vi "CS SQL Server.queryOneStr.vi"(8 "error in (no error)":errorcluster, 10 "SQL query":string, 11 "connection reference":T1) -> (0 "error out":errorcluster, 1 "Query result":string, 3 "connection reference out":T1)   [LabVIEW 2014, in "CS SQL Server.lvlib"]
doc: "Thisa VI executes a SQL statement.\n\nIt is assumed that this quey expectes one element as result only!"
uses:
  CS SQL Server.lvlib
  <vilib>/addons/database/Connection.llb/Conn ObjectReference.ctl
  <vilib>/addons/database/Recordset.llb/Rec Destroy - Connection.vi
  <vilib>/addons/database/Recordset.llb/Rec Fetch Recordset Data (R).vi
  <vilib>/addons/database/Connection.llb/Conn Execute.vi
  <vilib>/addons/database/_DB Variant To Data/Database Variant To Data.xnode
  <vilib>/addons/database/NI_Database_API.lvlib
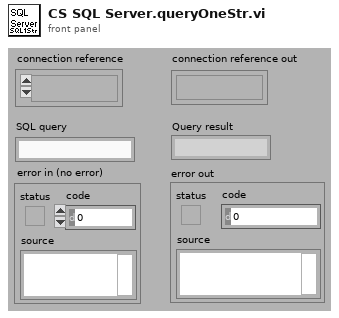
[diagram p1: front panel]
types:
  T1 = typedef "NI_Database_API.lvlib/Conn ObjectReference.ctl" = refnum<k1>
  T2 = typedef "NI_Database_API.lvlib/Rec ObjectReference.ctl" = refnum<k1>
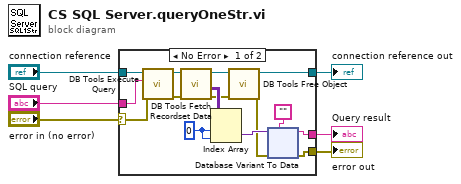
[diagram p0: block diagram]
diagram:
  n1 = case shown="No Error" "error in (no error)" {
    selector: "error in (no error)" -> [w7 w54]
    tunnel: "connection reference" -> [w12 w55]
    tunnel: "SQL query" -> [w11 _]
    tunnel: [w10 w55] -> w4
    tunnel: [w9 _] -> w3
    tunnel: [w8 w54] -> w2
    frame No Error {
      w21 = 0 ("Index (row)")
      n2 = call-poly <vilib>:"DB Tools Execute Query.vi"("error in (no error)"=w7, "SQL query"=w11, "connection reference"=w12) -> ("error out"=w20:errorcluster, "recordset reference"=w19:T2)  [unwired: 5 in]
      n3 = call-poly <vilib>:"DB Tools Fetch Recordset Data.vi"("error in (no error)"=w20, "recordset reference"=w19) -> ("error out"=w17:errorcluster, "recordset data"=w18:variant[][], "recordset reference out"=w16:T2)  [unwired: 3 in]
      n4 = Index Array(array=w18, index (row)=w21, index (col)=w21) -> (element=w15:variant)
      n5 = call-poly <vilib>:"DB Tools Free Object.vi"("error in (no error)"=w17, "recordset reference"=w16) -> ("error out"=w13:errorcluster, "connection reference"=w10:T1)  [unwired: 8 in]
      n6 = xnode "Database Variant To Data"("database variant"=w15, "error in (no error)"=w13, "type"="") -> ("data"=w9:string, "error out"=w8:errorcluster)
    }
    frame Error {
    }
  }
  "connection reference out" <- w4
  "Query result" <- w3
  "error out" <- w2
